vi "SunplusDailyS2T.vi"() -> ()   [LabVIEW 2012]
uses:
  <vilib>/addons/database/Auxilliary.llb/DB Tools Cursor Type.ctl
  <vilib>/Utility/NIReport.llb/NI_report.lvclass
  <vilib>/addons/database/Connection.llb/DB Tools Open Connec (Path).vi
  <vilib>/addons/database/Connection.llb/Conn Execute.vi
  <vilib>/addons/database/Recordset.llb/Rec Fetch Recordset Data (R).vi
  <vilib>/addons/database/Recordset.llb/Rec Destroy - Connection.vi
  <vilib>/addons/database/_DB Variant To Data/Database Variant To Data.xnode
  <vilib>/addons/database/NI_Database_API.lvlib
  <vilib>/Utility/NIReport.llb/Excel/NI_Excel.lvclass
  <vilib>/Utility/SMTP/NI_SMTPEmail.lvlib
panel:
  in  "start (0, 0) 2":cluster{"start row":i32, "start column":i32}
  out "error out 2":errorcluster
  in  "MIME content-type (application/octet-stream)":string="application/octet-stream"
  out "error out 4":errorcluster
  in  "?":cluster{"start row":i32, "start column":i32}
  out "error out":errorcluster
  in  "start (0, 0)":cluster{"start row":i32, "start column":i32}
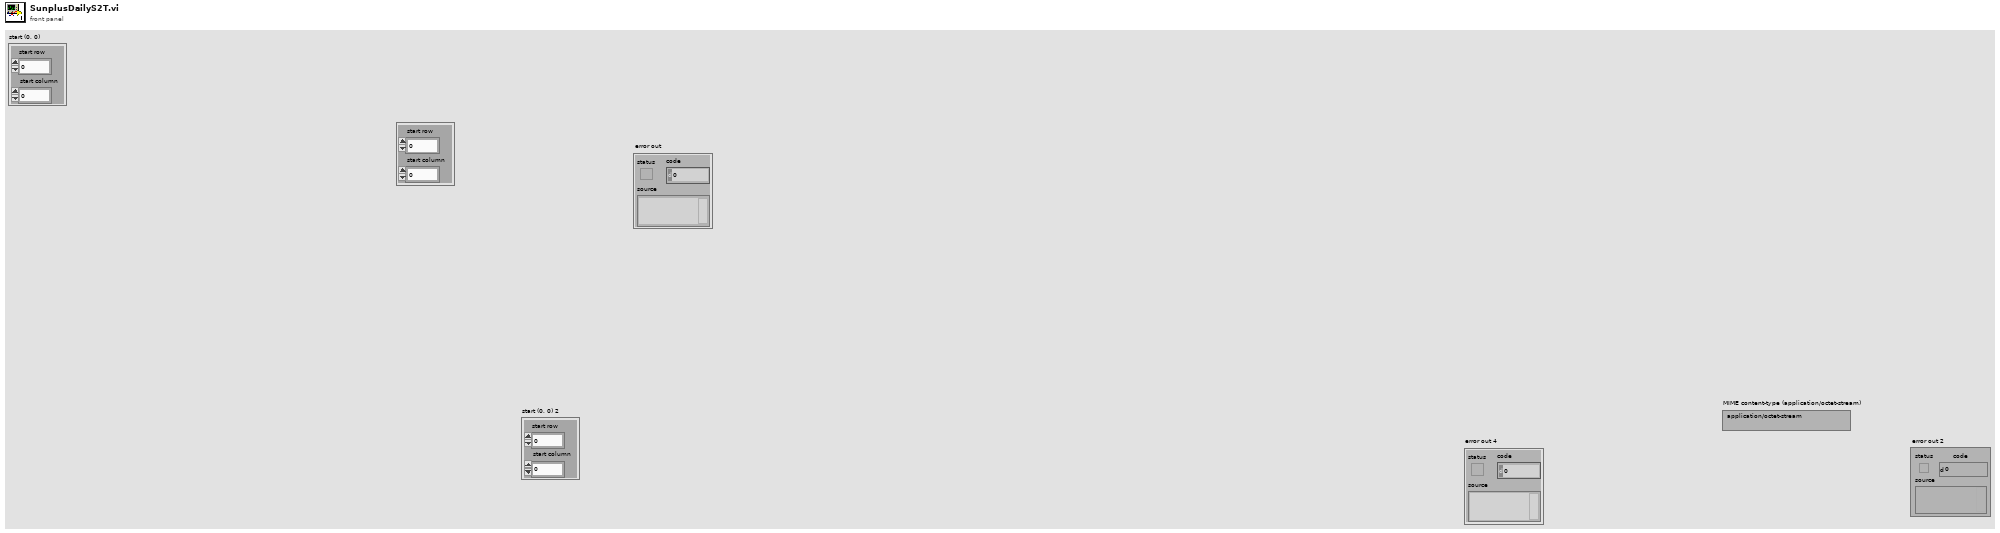
[diagram p1: front panel]
types:
  T1 = typedef "NI_Database_API.lvlib/DB Tools Cursor Type.ctl" = enum16{"forward-only", "keyset", "dynamic", "static"}
  T2 = enum16{"Standard Report", "HTML", "Word", "Excel"}
  T3 = typedef "NI_Database_API.lvlib/Conn ObjectReference.ctl" = refnum<k1>
  T4 = typedef "NI_Database_API.lvlib/Rec ObjectReference.ctl" = refnum<k1>
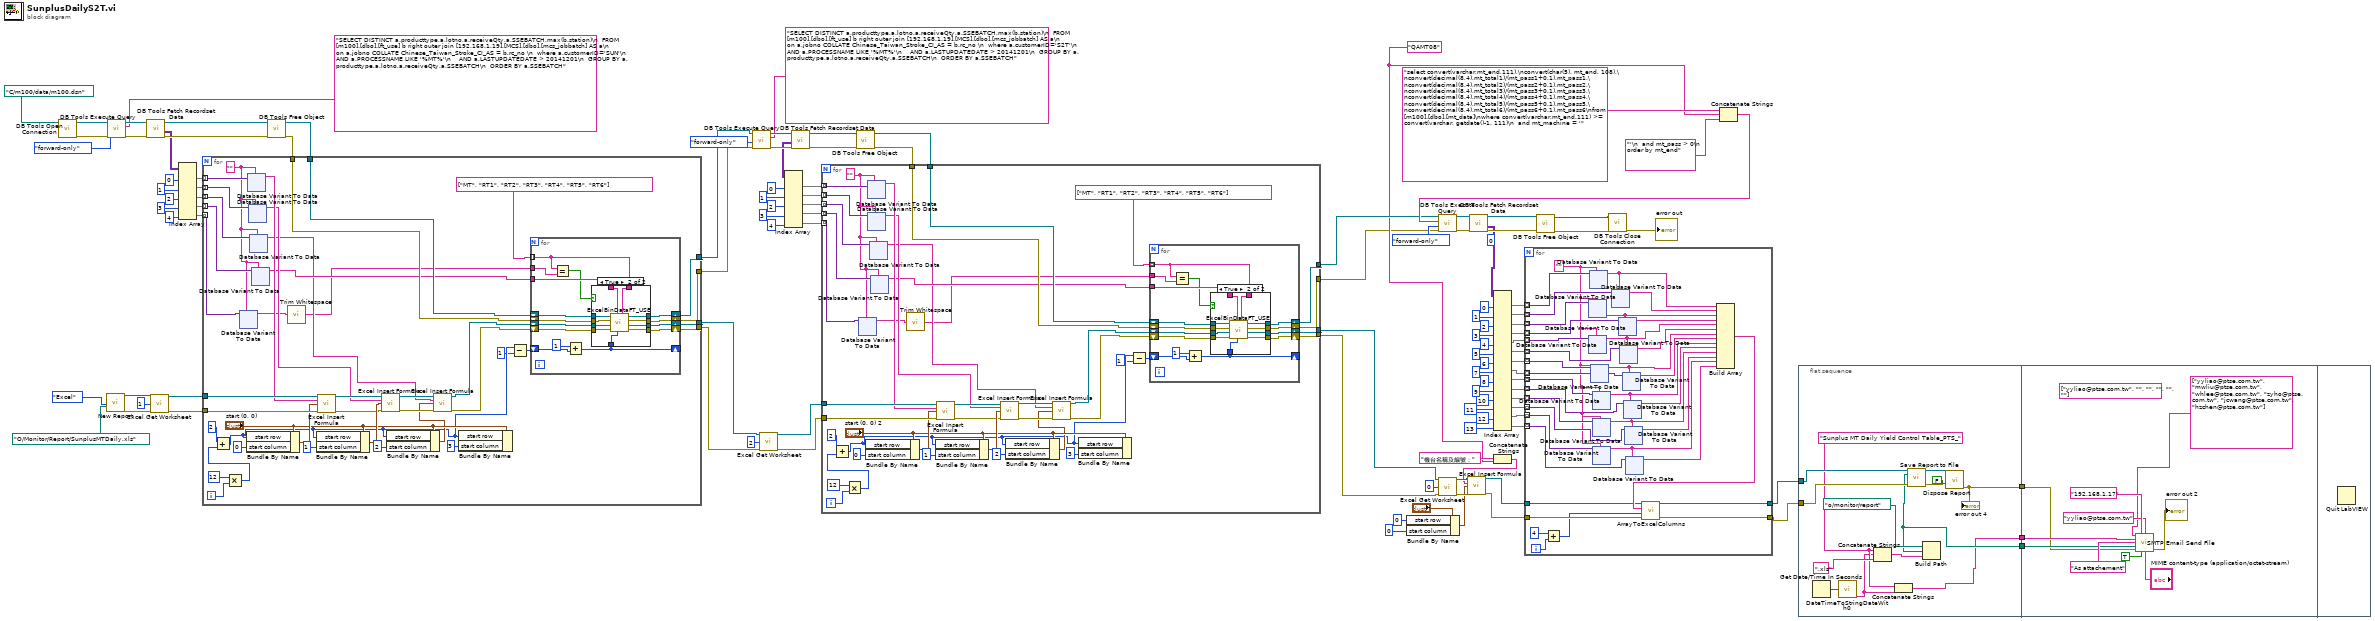
[diagram p0: block diagram]
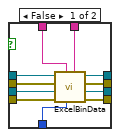
[diagram p2: hidden frame]
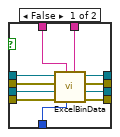
[diagram p3: hidden frame]
diagram:
  w2 = "QAMT08" ("Machine")
  (unwired) 0 ("index")
  n1 = call-poly <vilib>:"DB Tools Open Connection.vi"("connection information"=path "C:/m100/data/m100.dsn") -> ("error out"=w108:errorcluster, "connection reference"=w109:T3)  [unwired: 7 in]
  n2 = call <vilib>:"New Report.vi"("report type"=T2."Excel" ("Report Type"), "template (empty)"=path "O:/Monitor/Report/SunplusMTDaily.xls") -> ("report out"=w93:refnum<class "NI_report.lvclass">, "error out"=w92:errorcluster)  [unwired: 12 in]
  n3 = call-poly <vilib>:"DB Tools Execute Query.vi"("error in (no error)"=w108, "cursor type"=DB_Tools_Cursor_Type."forward-only", "SQL query"="SELECT DISTINCT a.producttype,a.lotno,a.receiveQty,a.SSEBATCH,max(b.station)\n  FROM [m100].[dbo].[ft_use] b right outer join [192.168.1.19].[MCS].[dbo].[mcs_jobbatch] AS a\n  on a.jobno COLLATE Chinese_Taiwan_Stroke_CI_AS = b.rc_no \n  where a.customerID='SUN'\n    AND a.PROCESSNAME LIKE '%MT%'\n    AND a.LASTUPDATEDATE > 20141201\n  GROUP BY a.producttype,a.lotno,a.receiveQty,a.SSEBATCH\n  ORDER BY a.SSEBATCH", "connection reference"=w109) -> ("error out"=w110:errorcluster, "recordset reference"=w111:T4)  [unwired: 4 in]
  n4 = call-poly <vilib>:"DB Tools Fetch Recordset Data.vi"("error in (no error)"=w110, "recordset reference"=w111) -> ("error out"=w112:errorcluster, "recordset data"=w105:variant[][], "recordset reference out"=w113:T4)  [unwired: 3 in]
  n5 = call <vilib>:"Excel Get Worksheet.vi"("report in"=w93, "worksheet index (0)"=1, "error in (no error)"=w92) -> ("report out"=w89:refnum<class "NI_report.lvclass">, "error out"=w88:errorcluster)  [unwired: 11 in]
  n6 = Index Array(array=w105, index (col) #1=0 ("disabled index (col)"), index (col) #2=1 ("index (col)"), index (col) #3=2 ("index (col)"), index (col) #4=3 ("index (col)"), index (col) #5=4 ("index (col)")) -> (element #1=w101:variant[], element #2=w100:variant[], element #3=w99:variant[], element #4=w95:variant[], element #5=w32:variant[])  [unwired: 5 in]
  n7 = call-poly <vilib>:"DB Tools Free Object.vi"("error in (no error)"=w112, "recordset reference"=w113) -> ("error out"=w98:errorcluster, "connection reference"=w97:T3)  [unwired: 8 in]
  n8 = for {
    tunnel: w101 -> [w158] mode=indexing
    tunnel: w100 -> [w157] mode=indexing
    tunnel: w99 -> [w156] mode=indexing
    tunnel: w98 -> [w133]
    tunnel: w97 -> [w134]
    tunnel: w95 -> [w155] mode=indexing
    tunnel: w89 -> [w154]
    tunnel: w88 -> [w153]
    tunnel: [w124] -> w8
    tunnel: [w123] -> w7
    tunnel: [w126] -> w26
    tunnel: [w125] -> w25
    tunnel: w32 -> [w120] mode=indexing
    i -> [w137]
    w119 = ""
    n9 = Multiply(x=12, y=w137) -> (x*y=w135:i32)
    n10 = Add(x=2, y=w135) -> (x+y=w130:i32)
    n11 = xnode "Database Variant To Data"("database variant"=w120, "type"=w119) -> ("data"=w118:string)  [unwired: 1 in, 1 out]
    n12 = Bundle By Name(cluster="start (0, 0)", "start row"=w130, "start column"=0) -> (w152:cluster{"start row":i32, "start column":i32})
    n13 = xnode "Database Variant To Data"("database variant"=w158, "type"=w119) -> ("data"=w149:string)  [unwired: 1 in, 1 out]
    n14 = xnode "Database Variant To Data"("database variant"=w157, "type"=w119) -> ("data"=w144:string)  [unwired: 1 in, 1 out]
    n15 = xnode "Database Variant To Data"("database variant"=w156, "type"=w119) -> ("data"=w121:string)  [unwired: 1 in, 1 out]
    n16 = xnode "Database Variant To Data"("database variant"=w155, "type"=w119) -> ("data"=w127:string)  [unwired: 1 in, 1 out]
    n17 = call <vilib>:"Trim Whitespace.vi"("string"=w118) -> ("trimmed string"=w117:string)  [unwired: 1 in]
    n18 = Bundle By Name(cluster="start (0, 0)", "start row"=w130, "start column"=1) -> (w147:cluster{"start row":i32, "start column":i32})
    n19 = call <vilib>:"Excel Insert Formula.vi"("report in"=w154, "formula"=w149, "start (0, 0)"=w152, "error in (no error)"=w153) -> ("report out"=w146:refnum<class "NI_report.lvclass">, "error out"=w145:errorcluster)  [unwired: 10 in]
    n20 = call <vilib>:"Excel Insert Formula.vi"("report in"=w146, "formula"=w144, "start (0, 0)"=w147, "error in (no error)"=w145) -> ("report out"=w142:refnum<class "NI_report.lvclass">, "error out"=w141:errorcluster)  [unwired: 10 in]
    n21 = Bundle By Name(cluster="start (0, 0)", "start row"=w130, "start column"=2) -> (w138:cluster{"start row":i32, "start column":i32})
    n22 = call <vilib>:"Excel Insert Formula.vi"("report in"=w142, "formula"=w121, "start (0, 0)"=w138, "error in (no error)"=w141) -> ("report out"=w132:refnum<class "NI_report.lvclass">, "error out"=w131:errorcluster)  [unwired: 10 in]
    n23 = Bundle By Name(cluster="start (0, 0)", "start row"=w130, "start column"=3) -> ()  [unwired: 1 out]
    n24 = Subtract(x=w130, y=1) -> (x-y=w128:i32)
    n25 = for {
      shift-right: [w204] -> w126
      shift-left: w134 -> [w197]
      shift-right: [w203] -> w125
      shift-left: w133 -> [w196]
      shift-right: [w202] -> w124
      shift-left: w132 -> [w195]
      shift-right: [w201] -> w123
      shift-left: w131 -> [w194]
      shift-right: [w200] -> _
      shift-left: w128 -> [w199]
      tunnel: w127 -> [w198]
      tunnel: string[] ["MT", "RT1", "RT2", "RT3", "RT4", "RT5", "RT6"] ("Array") -> [w192] mode=indexing
      tunnel: w117 -> [w193]
      n26 = Equal?(x=w192, y=w193) -> (x = y?=w191:bool)
      n27 = Add(x=1, y=w199) -> (x+y=w200:i32)
      n28 = case shown="True" w191 {
        tunnel: [w216 w222] -> w204
        tunnel: [w215 w221] -> w203
        tunnel: [w214 w220] -> w202
        tunnel: [w213 w219] -> w201
        tunnel: w200 -> [w212 w227]
        tunnel: w198 -> [w211 w218]
        tunnel: w197 -> [w210 w226]
        tunnel: w196 -> [w209 w225]
        tunnel: w195 -> [w208 w224]
        tunnel: w194 -> [w207 w223]
        tunnel: w192 -> [w206 w217]
        frame False {
          n29 = call "ExcelBinData.vi"("step"=w206, "start row"=w212, "jobno"=w211, "error in (no error) 2"=w207, "report in"=w208, "error in (no error)"=w209, "connection reference 2"=w210) -> ("error out 2"=w213:errorcluster, "report out"=w214:refnum<class "NI_report.lvclass">, "error out"=w215:errorcluster, "connection reference"=w216:T3)  [unwired: 1 in]
        }
        frame True {
          n30 = call "ExcelBinDataFT_USE.vi"("step"=w217, "start row"=w227, "jobno"=w218, "error in (no error) 2"=w223, "report in"=w224, "error in (no error)"=w225, "connection reference 2"=w226) -> ("error out 2"=w219:errorcluster, "report out"=w220:refnum<class "NI_report.lvclass">, "error out"=w221:errorcluster, "connection reference"=w222:T3)  [unwired: 1 in]
        }
      }
    }
  }
  n31 = call-poly <vilib>:"DB Tools Execute Query.vi"("error in (no error)"=w25, "cursor type"=DB_Tools_Cursor_Type."forward-only", "SQL query"="SELECT DISTINCT a.producttype,a.lotno,a.receiveQty,a.SSEBATCH,max(b.station)\n  FROM [m100].[dbo].[ft_use] b right outer join [192.168.1.19].[MCS].[dbo].[mcs_jobbatch] AS a\n  on a.jobno COLLATE Chinese_Taiwan_Stroke_CI_AS = b.rc_no \n  where a.customerID='S2T'\n    AND a.PROCESSNAME LIKE '%MT%'\n    AND a.LASTUPDATEDATE > 20141201\n  GROUP BY a.producttype,a.lotno,a.receiveQty,a.SSEBATCH\n  ORDER BY a.SSEBATCH", "connection reference"=w26) -> ("error out"=w28:errorcluster, "recordset reference"=w29:T4)  [unwired: 4 in]
  n32 = call <vilib>:"Excel Get Worksheet.vi"("report in"=w8, "worksheet index (0)"=2, "error in (no error)"=w7) -> ("report out"=w10:refnum<class "NI_report.lvclass">, "error out"=w9:errorcluster)  [unwired: 11 in]
  n33 = call-poly <vilib>:"DB Tools Fetch Recordset Data.vi"("error in (no error)"=w28, "recordset reference"=w29) -> ("error out"=w30:errorcluster, "recordset data"=w19:variant[][], "recordset reference out"=w31:T4)  [unwired: 3 in]
  n34 = Index Array(array=w19, index (col) #1=0 ("disabled index (col)"), index (col) #2=1 ("index (col)"), index (col) #3=2 ("index (col)"), index (col) #4=3 ("index (col)"), index (col) #5=4 ("index (col)")) -> (element #1=w17:variant[], element #2=w16:variant[], element #3=w15:variant[], element #4=w14:variant[], element #5=w13:variant[])  [unwired: 5 in]
  n35 = call-poly <vilib>:"DB Tools Free Object.vi"("error in (no error)"=w30, "recordset reference"=w31) -> ("error out"=w12:errorcluster, "connection reference"=w11:T3)  [unwired: 8 in]
  n36 = for {
    tunnel: w17 -> [w397] mode=indexing
    tunnel: w16 -> [w396] mode=indexing
    tunnel: w15 -> [w395] mode=indexing
    tunnel: w12 -> [w372]
    tunnel: w11 -> [w373]
    tunnel: w14 -> [w394] mode=indexing
    tunnel: w10 -> [w393]
    tunnel: w9 -> [w392]
    tunnel: [w363] -> w5
    tunnel: [w362] -> w4
    tunnel: [w365] -> w3
    tunnel: [w364] -> w1
    tunnel: w13 -> [w359] mode=indexing
    i -> [w376]
    w358 = ""
    n37 = Multiply(x=12, y=w376) -> (x*y=w374:i32)
    n38 = Add(x=2, y=w374) -> (x+y=w369:i32)
    n39 = xnode "Database Variant To Data"("database variant"=w359, "type"=w358) -> ("data"=w357:string)  [unwired: 1 in, 1 out]
    n40 = Bundle By Name(cluster="start (0, 0) 2", "start row"=w369, "start column"=0) -> (w391:cluster{"start row":i32, "start column":i32})
    n41 = xnode "Database Variant To Data"("database variant"=w397, "type"=w358) -> ("data"=w388:string)  [unwired: 1 in, 1 out]
    n42 = xnode "Database Variant To Data"("database variant"=w396, "type"=w358) -> ("data"=w383:string)  [unwired: 1 in, 1 out]
    n43 = xnode "Database Variant To Data"("database variant"=w395, "type"=w358) -> ("data"=w360:string)  [unwired: 1 in, 1 out]
    n44 = xnode "Database Variant To Data"("database variant"=w394, "type"=w358) -> ("data"=w366:string)  [unwired: 1 in, 1 out]
    n45 = call <vilib>:"Trim Whitespace.vi"("string"=w357) -> ("trimmed string"=w356:string)  [unwired: 1 in]
    n46 = Bundle By Name(cluster="start (0, 0) 2", "start row"=w369, "start column"=1) -> (w386:cluster{"start row":i32, "start column":i32})
    n47 = call <vilib>:"Excel Insert Formula.vi"("report in"=w393, "formula"=w388, "start (0, 0)"=w391, "error in (no error)"=w392) -> ("report out"=w385:refnum<class "NI_report.lvclass">, "error out"=w384:errorcluster)  [unwired: 10 in]
    n48 = call <vilib>:"Excel Insert Formula.vi"("report in"=w385, "formula"=w383, "start (0, 0)"=w386, "error in (no error)"=w384) -> ("report out"=w381:refnum<class "NI_report.lvclass">, "error out"=w380:errorcluster)  [unwired: 10 in]
    n49 = Bundle By Name(cluster="start (0, 0) 2", "start row"=w369, "start column"=2) -> (w377:cluster{"start row":i32, "start column":i32})
    n50 = call <vilib>:"Excel Insert Formula.vi"("report in"=w381, "formula"=w360, "start (0, 0)"=w377, "error in (no error)"=w380) -> ("report out"=w371:refnum<class "NI_report.lvclass">, "error out"=w370:errorcluster)  [unwired: 10 in]
    n51 = Bundle By Name(cluster="start (0, 0) 2", "start row"=w369, "start column"=3) -> ()  [unwired: 1 out]
    n52 = Subtract(x=w369, y=1) -> (x-y=w367:i32)
    n53 = for {
      shift-right: [w443] -> w365
      shift-left: w373 -> [w436]
      shift-right: [w442] -> w364
      shift-left: w372 -> [w435]
      shift-right: [w441] -> w363
      shift-left: w371 -> [w434]
      shift-right: [w440] -> w362
      shift-left: w370 -> [w433]
      shift-right: [w439] -> _
      shift-left: w367 -> [w438]
      tunnel: w366 -> [w437]
      tunnel: string[] ["MT", "RT1", "RT2", "RT3", "RT4", "RT5", "RT6"] ("Array") -> [w431] mode=indexing
      tunnel: w356 -> [w432]
      n54 = Equal?(x=w431, y=w432) -> (x = y?=w430:bool)
      n55 = Add(x=1, y=w438) -> (x+y=w439:i32)
      n56 = case shown="True" w430 {
        tunnel: [w455 w461] -> w443
        tunnel: [w454 w460] -> w442
        tunnel: [w453 w459] -> w441
        tunnel: [w452 w458] -> w440
        tunnel: w439 -> [w451 w466]
        tunnel: w437 -> [w450 w457]
        tunnel: w436 -> [w449 w465]
        tunnel: w435 -> [w448 w464]
        tunnel: w434 -> [w447 w463]
        tunnel: w433 -> [w446 w462]
        tunnel: w431 -> [w445 w456]
        frame False {
          n57 = call "ExcelBinData.vi"("step"=w445, "start row"=w451, "jobno"=w450, "error in (no error) 2"=w446, "report in"=w447, "error in (no error)"=w448, "connection reference 2"=w449) -> ("error out 2"=w452:errorcluster, "report out"=w453:refnum<class "NI_report.lvclass">, "error out"=w454:errorcluster, "connection reference"=w455:T3)  [unwired: 1 in]
        }
        frame True {
          n58 = call "ExcelBinDataFT_USE.vi"("step"=w456, "start row"=w466, "jobno"=w457, "error in (no error) 2"=w462, "report in"=w463, "error in (no error)"=w464, "connection reference 2"=w465) -> ("error out 2"=w458:errorcluster, "report out"=w459:refnum<class "NI_report.lvclass">, "error out"=w460:errorcluster, "connection reference"=w461:T3)  [unwired: 1 in]
        }
      }
    }
  }
  n59 = Bundle By Name(cluster="?", "start row"=0, "start column"=0) -> (w41:cluster{"start row":i32, "start column":i32})
  n60 = call <vilib>:"Excel Get Worksheet.vi"("report in"=w5, "worksheet index (0)"=0, "error in (no error)"=w4) -> ("report out"=w46:refnum<class "NI_report.lvclass">, "error out"=w45:errorcluster)  [unwired: 11 in]
  n61 = Concatenate Strings("機台名稱及編號：" ("formula"), w2) -> (w38:string)
  n62 = call <vilib>:"Excel Insert Formula.vi"("report in"=w46, "formula"=w38, "start (0, 0)"=w41, "error in (no error)"=w45) -> ("report out"=w40:refnum<class "NI_report.lvclass">, "error out"=w39:errorcluster)  [unwired: 10 in]
  n63 = Concatenate Strings("select convert(varchar,mt_end,111),\nconvert(char(5), mt_end, 108),\nconvert(decimal(8,4),mt_total1)/(mt_pass1+0.1),mt_pass1,\nconvert(decimal(8,4),mt_total2)/(mt_pass2+0.1),mt_pass2,\nconvert(decimal(8,4),mt_total3)/(mt_pass3+0.1),mt_pass3,\nconvert(decimal(8,4),mt_total4)/(mt_pass4+0.1),mt_pass4,\nconvert(decimal(8,4),mt_total5)/(mt_pass5+0.1),mt_pass5,\nconvert(decimal(8,4),mt_total6)/(mt_pass6+0.1),mt_pass6\nfrom [m100].[dbo].[mt_data]\nwhere convert(varchar,mt_end,111) >= convert(varchar, getdate()-1, 111)\n  and mt_machine = '" ("SQL query"), w2, "'\n  and mt_pass > 0\n  order by mt_end" ("SQL query")) -> (w47:string)
  n64 = call-poly <vilib>:"DB Tools Execute Query.vi"("error in (no error)"=w1, "cursor type"=DB_Tools_Cursor_Type."forward-only", "SQL query"=w47, "connection reference"=w3) -> ("error out"=w86:errorcluster, "recordset reference"=w85:T4)  [unwired: 4 in]
  n65 = call-poly <vilib>:"DB Tools Fetch Recordset Data.vi"("error in (no error)"=w86, "recordset reference"=w85) -> ("error out"=w83:errorcluster, "recordset data"=w78:variant[][], "recordset reference out"=w84:T4)  [unwired: 3 in]
  n66 = Index Array(array=w78, index (col) #1=0 ("disabled index (col)"), index (col) #2=1 ("index (col)"), index (col) #3=2 ("index (col)"), index (col) #4=3 ("index (col)"), index (col) #5=4 ("index (col)"), index (col) #6=5 ("index (col)"), index (col) #7=6 ("index (col)"), index (col) #8=7 ("index (col)"), index (col) #9=8 ("index (col)"), index (col) #10=9 ("index (col)"), index (col) #11=10 ("index (col)"), index (col) #12=11 ("index (col)"), index (col) #13=12 ("index (col)"), index (col) #14=13 ("index (col)")) -> (element #1=w75:variant[], element #2=w74:variant[], element #3=w73:variant[], element #4=w62:variant[], element #5=w61:variant[], element #6=w60:variant[], element #7=w59:variant[], element #8=w58:variant[], element #9=w57:variant[], element #10=w56:variant[], element #11=w55:variant[], element #12=w54:variant[], element #13=w51:variant[], element #14=w50:variant[])  [unwired: 14 in]
  n67 = for {
    tunnel: w75 -> [w631] mode=indexing
    tunnel: w74 -> [w630] mode=indexing
    tunnel: w73 -> [w629] mode=indexing
    tunnel: w62 -> [w627] mode=indexing
    tunnel: w61 -> [w623] mode=indexing
    tunnel: w60 -> [w621] mode=indexing
    tunnel: w59 -> [w619] mode=indexing
    tunnel: w58 -> [w616] mode=indexing
    tunnel: w57 -> [w615] mode=indexing
    tunnel: w56 -> [w614] mode=indexing
    tunnel: w55 -> [w611] mode=indexing
    tunnel: w54 -> [w610] mode=indexing
    tunnel: w51 -> [w607] mode=indexing
    tunnel: w50 -> [w606] mode=indexing
    tunnel: w40 -> [w601]
    tunnel: w39 -> [w600]
    tunnel: [w596] -> w36
    tunnel: [w595] -> w35
    i -> [w599]
    w603 = ""
    n68 = Add(x=4, y=w599) -> (x+y=w597:i32)
    n69 = xnode "Database Variant To Data"("database variant"=w629, "type"=w603) -> ("data"=w625:string)  [unwired: 1 in, 1 out]
    n70 = xnode "Database Variant To Data"("database variant"=w623, "type"=w603) -> ("data"=w622:string)  [unwired: 1 in, 1 out]
    n71 = xnode "Database Variant To Data"("database variant"=w631, "type"=w603) -> ("data"=w626:string)  [unwired: 1 in, 1 out]
    n72 = xnode "Database Variant To Data"("database variant"=w619, "type"=w603) -> ("data"=w618:string)  [unwired: 1 in, 1 out]
    n73 = xnode "Database Variant To Data"("database variant"=w615, "type"=w603) -> ("data"=w613:string)  [unwired: 1 in, 1 out]
    n74 = xnode "Database Variant To Data"("database variant"=w611, "type"=w603) -> ("data"=w609:string)  [unwired: 1 in, 1 out]
    n75 = xnode "Database Variant To Data"("database variant"=w607, "type"=w603) -> ("data"=w605:string)  [unwired: 1 in, 1 out]
    n76 = xnode "Database Variant To Data"("database variant"=w630, "type"=w626) -> ("data"=w628:string)  [unwired: 1 in, 1 out]
    n77 = xnode "Database Variant To Data"("database variant"=w627, "type"=w625) -> ("data"=w624:string)  [unwired: 1 in, 1 out]
    n78 = xnode "Database Variant To Data"("database variant"=w621, "type"=w622) -> ("data"=w620:string)  [unwired: 1 in, 1 out]
    n79 = xnode "Database Variant To Data"("database variant"=w616, "type"=w618) -> ("data"=w617:string)  [unwired: 1 in, 1 out]
    n80 = xnode "Database Variant To Data"("database variant"=w614, "type"=w613) -> ("data"=w612:string)  [unwired: 1 in, 1 out]
    n81 = xnode "Database Variant To Data"("database variant"=w610, "type"=w609) -> ("data"=w608:string)  [unwired: 1 in, 1 out]
    n82 = xnode "Database Variant To Data"("database variant"=w606, "type"=w605) -> ("data"=w604:string)  [unwired: 1 in, 1 out]
    n83 = Build Array(w626, w628, w625, w624, w622, w620, w618, w617, w613, w612, w609, w608, w605, w604) -> (w602:string[])
    n84 = call "ArrayToExcelColumns.vi"("error in (no error)"=w600, "start row"=w597, "ArrayData"=w602, "report in"=w601) -> ("error in (no error) 2"=w595:errorcluster, "report in 2"=w596:refnum<class "NI_report.lvclass">)  [unwired: 6 in]
  }
  n85 = call-poly <vilib>:"DB Tools Free Object.vi"("error in (no error)"=w83, "recordset reference"=w84) -> ("error out"=w81:errorcluster, "connection reference"=w82:T3)  [unwired: 8 in]
  n86 = call <vilib>:"DB Tools Close Connection.vi"("error in (no error)"=w81, "connection reference"=w82) -> ("error out"=→"error out":errorcluster)  [unwired: 5 in]
  n87 = flat-sequence {
    tunnel: w36 -> [w1089]
    tunnel: w35 -> [w1088]
    tunnel: [w1080] -> w116
    tunnel: [w1084] -> w115
    tunnel: [w1083] -> w114
    tunnel: w116 -> [w1097]
    tunnel: w115 -> [w1096]
    tunnel: w114 -> [w1095]
    frame #0 {
      w1082 = "Sunplus MT Daily Yield Control Table_PTS_" ("string")
      n88 = Get Date/Time In Seconds() -> (seconds since 1Jan1904=w1086:timestamp)
      n89 = call "DateTimeToStringDateWith0.vi"("time stamp"=w1086) -> ("Dateyyyymmdd"=w1081:string)  [unwired: 9 in, 1 out]
      n90 = Concatenate Strings(w1082, w1081, ".xls" ("string")) -> (w1085:string)
      n91 = Concatenate Strings(w1082, w1081) -> (w1080:string)
      n92 = Build Path(base path=path "o:/monitor/report", name or relative path=w1085) -> (appended path=w1084:path)
      n93 = call-dynamic "Save Report to File.vi"("report in"=w1089, "report file path"=w1084, "error in (no error)"=w1088) -> ("report out"=w1091:refnum<class "NI_report.lvclass">, "error out"=w1090:errorcluster)  [unwired: 11 in]
      n94 = call-dynamic "Dispose Report.vi"("report in"=w1091, "save changes? (F)"=FALSE, "error in (no error)"=w1090) -> ("error out"=w1083:errorcluster)  [unwired: 12 in]
      "error out 4" <- w1083
    }
    frame #1 {
      (unwired) string[] ["yyliao@ptse.com.tw", "", "", "", "", ""] ("recipients")
      n95 = call <vilib>:"SMTP Email Send File.vi"("recipients"=string[] ["yyliao@ptse.com.tw", "mwliu@ptse.com.tw", "whlee@ptse.com.tw", "zyho@ptse.com.tw", "jcwang@ptse.com.tw", "hzchen@ptse.com.tw"], "mail server"="192.168.1.17", "return address"="yyliao@ptse.com.tw", "subject ([No Subject])"=w1097, "message"="As attachement", "file path"=w1096, "error in (no error)"=w1095, "binary? (F)"=TRUE, "MIME content-type (application/octet-stream)"="MIME content-type (application/octet-stream)") -> ("error out"=→"error out 2":errorcluster)  [unwired: 5 in, 1 out]
    }
    frame #2 {
      n96 = Quit LabVIEW() -> ()  [unwired: 1 in]
    }
  }
